vi "plot_text_glitch_damaged.vi"(7 "D of clusters":cluster{"D_giltch":ext}[](array[cluster]), 9 "precision":i32, 10 "index":i32, 11 "array clusters":cluster{"giltch_coord":dbl[]}[](array[cluster])) -> (2 "string":string, 3 "Origin":cluster{"X":i32, "Y":i32})   [LabVIEW 2017]
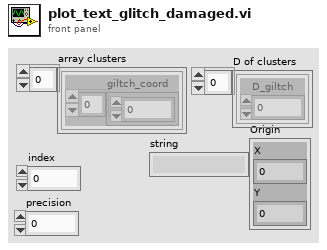
[diagram p1: front panel]
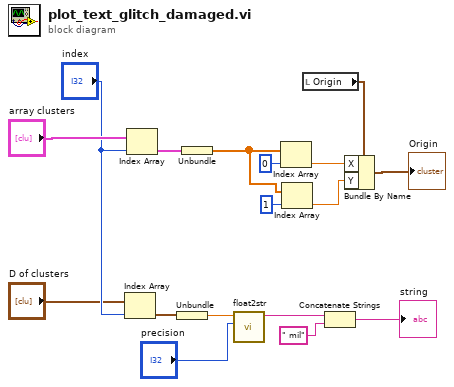
[diagram p0: block diagram]
diagram:
  n1 = Index Array(array="D of clusters", index="index") -> (element=w6:cluster{"D_giltch":ext})
  n2 = Index Array(array="array clusters", index="index") -> (element=w16:cluster{"giltch_coord":dbl[]})
  n3 = Unbundle(w6) -> ("D_giltch"=w5:ext)
  n4 = Unbundle(w16) -> ("giltch_coord"=w12:dbl[])
  n5 = call "float2str.vi"("precision"="precision", "float"=w5) -> ("string"=w3:string)  [unwired: 9 in]
  n6 = Index Array(array=w12, index=0) -> (element=w11:dbl)
  n7 = Index Array(array=w12, index=1) -> (element=w10:dbl)
  n8 = local read "Origin"() -> (w15:cluster{"X":i32, "Y":i32})
  n9 = Concatenate Strings(w3, " mil") -> (→"string":string)
  n10 = Bundle By Name(cluster=w15, "X"=w11, "Y"=w10) -> (→"Origin":cluster{"X":i32, "Y":i32})
